vi "Calculate power factor new version.vi"(5 "Dummy Vrms":dbl=120.0, 7 "error in":errorcluster, 8 "Use dummy Vout?":bool, 9 "InverterWaveforms":T1, 10 "Processing loop variables":T3 {"CurrInverter"."last updated" format="%<%H:%M\n%d/%m/%Y>T"; "CurrInverter"."set flag" items=["False", "True"]}) -> (0 "error out":errorcluster, 2 "InverterWaveforms":T1, 3 "Processing loop variables out":T3 {"CurrInverter"."last updated" format="%<%H:%M\n%d/%m/%Y>T"; "CurrInverter"."set flag" items=["False", "True"]})   [LabVIEW 2019, in "Main.lvclass"]
doc: "Developed by Kevin Thompson\nkevin@thompsonengineering.net\n\nCopyright 2020\nThompson Engineering, LLC"
uses:
  Main.lvclass
  Common/DataTypes/InverterWaveforms--cluster.ctl
  Common/DataTypes/ChannelWaveforms--cluster.ctl
  DataTypes/Processing loop variables--cluster.ctl
  DataTypes/averaging variables.ctl
  DataTypes/ESR alarm variables.ctl
  Common/DataTypes/Inverter database record v2--cluster.ctl
  Common/DataTypes/inverter info v2--cluster.ctl
  Common/DataTypes/inverter gain range--cluster.ctl
  Common/DataTypes/inverter offset range--cluster.ctl
  <vilib>/Analysis/NI_AALPro.lvlib
panel:
  # "time array is time in seconds at which samples are taken.\nSo for a 1000 HZ sample rate  0,  0.001, 0.002 .... \nneeded by nonlinear least square algorithm"
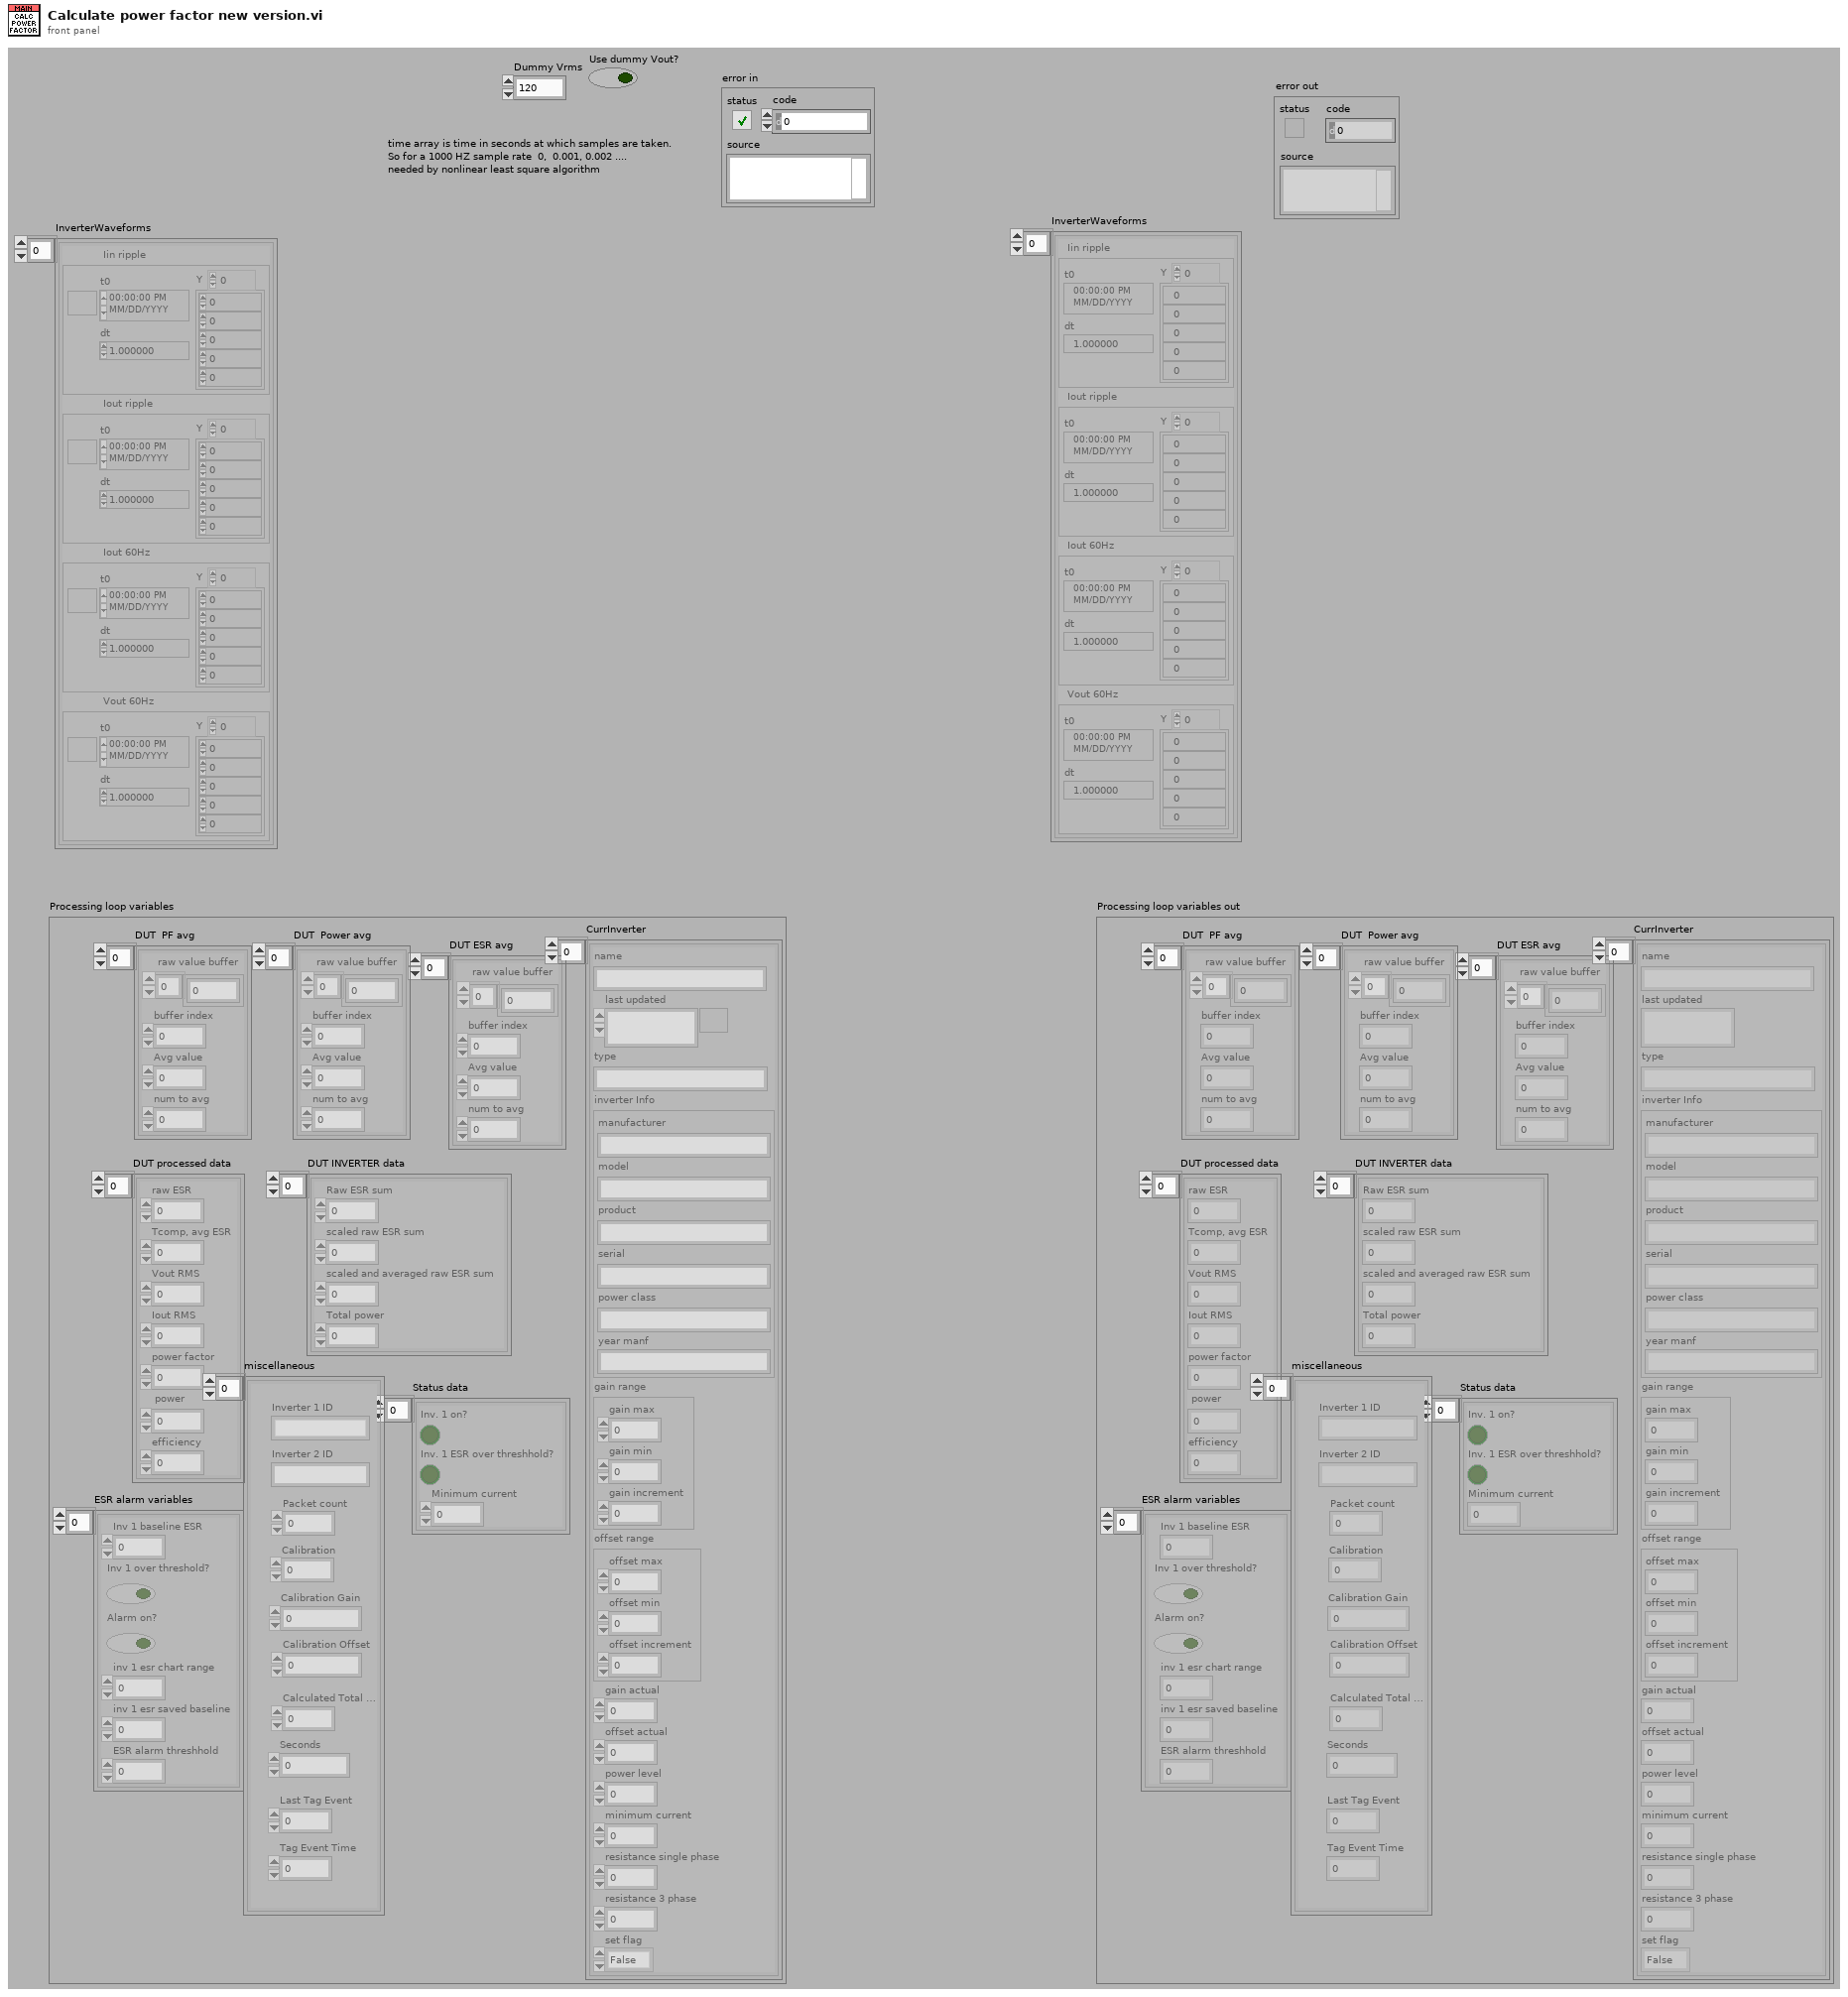
[diagram p1: front panel]
types:
  T1 = typedef "InverterWaveforms--cluster.ctl" = T2[]
  T2 = typedef "ChannelWaveforms--cluster.ctl" = cluster{"Iin ripple ":waveform(dbl), "Iout ripple ":waveform(dbl), "Iout 60Hz":waveform(dbl), "Vout 60Hz":waveform(dbl)}
  T3 = typedef "Main.lvclass/Processing loop variables--cluster.ctl" = cluster{"DUT ESR avg":T4[], "DUT  PF avg":T4[], "DUT  Power avg ":T4[], "DUT processed data":cluster{"raw ESR":dbl, "Tcomp, avg ESR":dbl, "Vout RMS":dbl, "Iout RMS":dbl, "power factor":dbl, "power":dbl, "efficiency":dbl}[], "ESR alarm variables":T5[], "Status data":cluster{"Inv. 1 on?":bool, "Inv. 1 ESR over threshhold?":bool, "Minimum current":dbl}[], "CurrInverter":T6[], "miscellaneous":cluster{"Inverter 1 ID":string, "Inverter 2 ID":string, "Packet count":u32, "Calibration":dbl, "Calibration Gain":dbl, "Calibration Offset":dbl, "Calculated Total Power":dbl, "Seconds":dbl, "Last Tag Event":dbl, "Tag Event Time":dbl}[], "DUT INVERTER data":cluster{"Raw ESR sum":dbl, "scaled raw ESR sum":dbl, "scaled and averaged raw ESR sum":dbl, "Total power":dbl}[]}
  T4 = typedef "Main.lvclass/averaging variables.ctl" = cluster{"raw value buffer":dbl[], "buffer index":i32, "Avg value":dbl, "num to avg":i32}
  T5 = typedef "Main.lvclass/ESR alarm variables.ctl" = cluster{"Inv 1 baseline ESR":dbl, "Inv 1 over threshold?":bool, "Alarm on?":bool, "inv 1 esr chart range":dbl, "inv 1 esr saved baseline":dbl, "ESR alarm threshhold":dbl}
  T6 = typedef "Inverter database record v2--cluster.ctl" = cluster{"name":string, "last updated":timestamp, "type":string, "inverter Info":T7, "gain range":T8, "offset range":T9, "gain actual":dbl, "offset actual":dbl, "power level":dbl, "minimum current":dbl, "resistance single phase":dbl, "resistance 3 phase":dbl, "set flag":u16}
  T7 = typedef "inverter info v2--cluster.ctl" = cluster{"manufacturer":string, "model":string, "product":string, "serial":string, "power class":string, "year manf":string}
  T8 = typedef "inverter gain range--cluster.ctl" = cluster{"gain max":dbl, "gain min":dbl, "gain increment":dbl}
  T9 = typedef "inverter offset range--cluster.ctl" = cluster{"offset max":dbl, "offset min":dbl, "offset increment":dbl}
  T10 = cluster{"raw ESR":dbl, "Tcomp, avg ESR":dbl, "Vout RMS":dbl, "Iout RMS":dbl, "power factor":dbl, "power":dbl, "efficiency":dbl}[]
  T11 = cluster{"Raw ESR sum":dbl, "scaled raw ESR sum":dbl, "scaled and averaged raw ESR sum":dbl, "Total power":dbl}[]
  T12 = cluster{"Power (Watts)":dbl, "Apparent Power (VA)":dbl, "Reactive Power (VAR)":dbl, "Power Factor":dbl}
  T13 = cluster{"raw ESR":dbl, "Tcomp, avg ESR":dbl, "Vout RMS":dbl, "Iout RMS":dbl, "power factor":dbl, "power":dbl, "efficiency":dbl}
  T14 = cluster{"Raw ESR sum":dbl, "scaled raw ESR sum":dbl, "scaled and averaged raw ESR sum":dbl, "Total power":dbl}
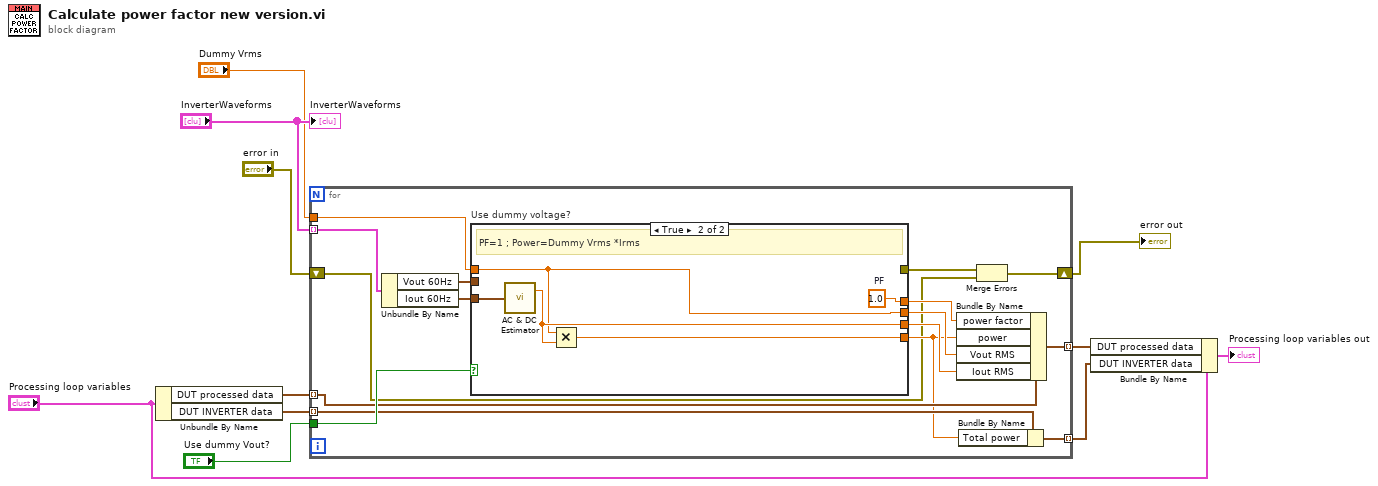
[diagram p0: block diagram]
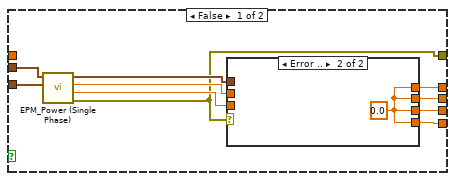
[diagram p2: hidden frame]
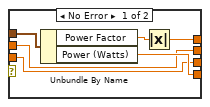
[diagram p3: hidden frame]
diagram:
  n1 = Unbundle By Name("Processing loop variables") -> ("DUT processed data"=w8:T10, "DUT INVERTER data"=w4:T11)
  n2 = for {
    tunnel: "InverterWaveforms" -> [w20] mode=indexing
    tunnel: "Use dummy Vout?" -> [w25]
    tunnel: "Dummy Vrms" -> [w21]
    tunnel: w8 -> [w19] mode=indexing
    tunnel: [w18] -> w6 mode=indexing
    tunnel: w4 -> [w17] mode=indexing
    tunnel: [w15] -> w3 mode=indexing
    shift-right: [w12] -> w1
    shift-left: "error in" -> [w14]
    n3 = Unbundle By Name(w20) -> ("Vout 60Hz"=w27:waveform(dbl), "Iout 60Hz"=w26:waveform(dbl))
    n4 = case "Use dummy voltage?" shown="True" w25 {
      tunnel: w27 -> [w37 _]
      tunnel: w26 -> [w36 w48]
      tunnel: [w31 w45] -> w23
      tunnel: [w29 w47] -> w22
      tunnel: [w34 w49] -> w16
      tunnel: [w33 w46] -> w24
      tunnel: w21 -> [_ w45]
      tunnel: [w28 _] -> w13
      frame False {
        n5 = call "EPM_Power (Single Phase).vi"("Current"=w36, "Voltage"=w37) -> ("error out"=w28:errorcluster, "Irms"=w30:dbl, "Vrms"=w32:dbl, "Power"=w35:T12)  [unwired: 6 in]
        n6 = case shown="Error .." w28 {
          tunnel: w35 -> [w43 _]
          tunnel: [w42 w44] -> w34
          tunnel: [w40 w44] -> w33
          tunnel: [w39 w44] -> w31
          tunnel: w32 -> [w39 _]
          tunnel: [w38 w44] -> w29
          tunnel: w30 -> [w38 _]
          frame No Error {
            n7 = Unbundle By Name(w43) -> ("Power Factor"=w41:dbl, "Power (Watts)"=w42:dbl)
            n8 = Absolute Value(x=w41) -> (abs(x)=w40:dbl)
          }
          frame Error {
            w44 = 0.0
          }
        }
      }
      frame True {
        w46 = 1.0  # PF
        # "PF=1 ; Power=Dummy Vrms *Irms"
        n9 = call <vilib>:"AC & DC Estimator.vi"("Signal (V)"=w48) -> ("AC estimate (Vrms)"=w47:dbl)  [unwired: 1 out]
        n10 = Multiply(x=w45, y=w47) -> (x*y=w49:dbl)
      }
    }
    n11 = Bundle By Name(cluster=w19, "power factor"=w24, "power"=w16, "Vout RMS"=w23, "Iout RMS"=w22) -> (w18:T13)
    n12 = Bundle By Name(cluster=w17, "Total power"=w16) -> (w15:T14)
    n13 = Merge Errors(w13, w14) -> (w12:errorcluster)
  }
  "error out" <- w1
  n14 = Bundle By Name(cluster="Processing loop variables", "DUT processed data"=w6, "DUT INVERTER data"=w3) -> (→"Processing loop variables out":T3)
  "InverterWaveforms" <- "InverterWaveforms"
